vi "NumberStringConv.vi"() -> ()   [LabVIEW 2012]
panel:
  out "Complete?":bool
  out "(remainder string)":string
  out "Numeric (dbl)":dbl
  in  "String":string
  out "Numeric (String %#g with %p)":dbl
  out "Numeric (%g) 2":dbl
  out "Numeric (%#g) 2":dbl
  out "Numeric (%p) 2":dbl
  out "Numeric (%#p) 2":dbl
  out "Numeric (%g)":dbl
  out "Numeric (%#g)":dbl
  out "Numeric (%p)":dbl
  out "Numeric (%#p)":dbl
  out "String (%#g)":string
  out "String (%g)":string
  out "String (%p)":string
  out "String (%#p)":string
  in  "Numeric (dbl)":dbl
  # "Frac/Exp String to Number"
  # "Scan Value"
  # "Summary: %#p is a nice way to get compact notation, but it must be \nundone with ScanValue.vi and %p format (which handles e-notation)!"
  # "And as shown at the left, the %p format with Scan Value will still take a\nscientific notation string back to a double correctly!"
  # "Try any input in this box to validate the conversion.\n(see block diagram for method)."
  # "- Try m/u/k/M notation\n- try scientific notation\n- try garbage like 34e9g"
  # "Can check for any remainder string to see if \nentire string used to make number."
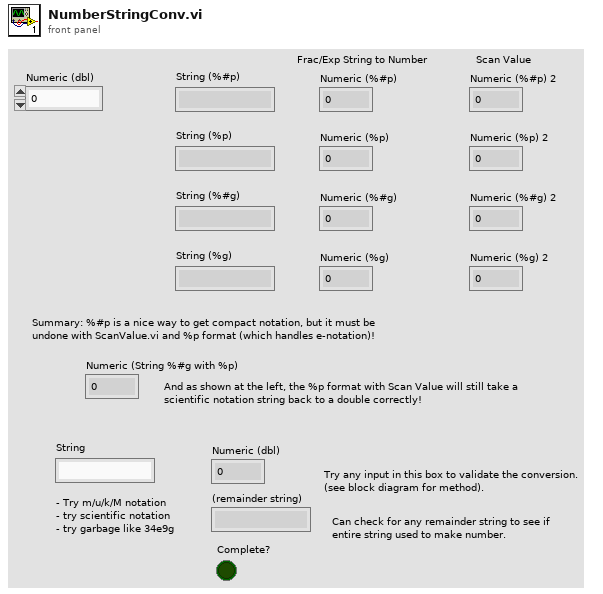
[diagram p1: front panel]
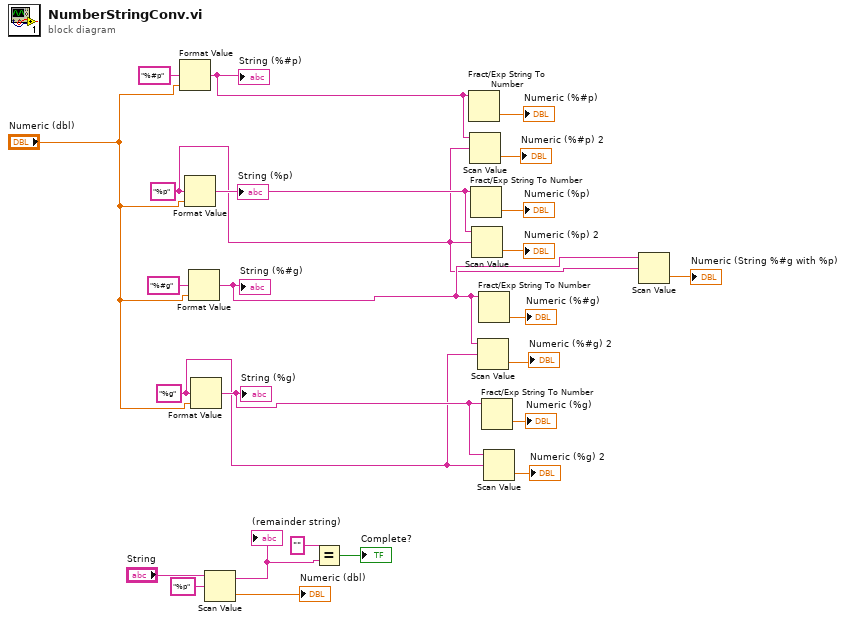
[diagram p0: block diagram]
diagram:
  w10 = "%g" ("format string")
  w7 = "%p" ("format string")
  n1 = Format Value(format string="%#p", value (0)="Numeric (dbl)") -> (output string=w15:string)  [unwired: 1 in]
  "String (%#p)" <- w15
  n2 = Format Value(format string=w7, value (0)="Numeric (dbl)") -> (output string=w14:string)  [unwired: 1 in]
  "String (%p)" <- w14
  n3 = Format Value(format string="%#g", value (0)="Numeric (dbl)") -> (output string=w8:string)  [unwired: 1 in]
  "String (%#g)" <- w8
  n4 = Format Value(format string=w10, value (0)="Numeric (dbl)") -> (output string=w13:string)  [unwired: 1 in]
  "String (%g)" <- w13
  n5 = Scan Value(string="String", format string="%p") -> (output string=w4:string, value=→"Numeric (dbl)":dbl)  [unwired: 1 in]
  "(remainder string)" <- w4
  n6 = Equal?(x="", y=w4) -> (x = y?=→"Complete?":bool)
  n7 = Fract/Exp String To Number(string=w15) -> (number=→"Numeric (%#p)":dbl)  [unwired: 3 in, 1 out]
  n8 = Scan Value(string=w15, format string=w7) -> (value=→"Numeric (%#p) 2":dbl)  [unwired: 1 in, 1 out]
  n9 = Fract/Exp String To Number(string=w14) -> (number=→"Numeric (%p)":dbl)  [unwired: 3 in, 1 out]
  n10 = Scan Value(string=w14, format string=w7) -> (value=→"Numeric (%p) 2":dbl)  [unwired: 1 in, 1 out]
  n11 = Scan Value(string=w8, format string=w10) -> (value=→"Numeric (%#g) 2":dbl)  [unwired: 1 in, 1 out]
  n12 = Fract/Exp String To Number(string=w8) -> (number=→"Numeric (%#g)":dbl)  [unwired: 3 in, 1 out]
  n13 = Fract/Exp String To Number(string=w13) -> (number=→"Numeric (%g)":dbl)  [unwired: 3 in, 1 out]
  n14 = Scan Value(string=w13, format string=w10) -> (value=→"Numeric (%g) 2":dbl)  [unwired: 1 in, 1 out]
  n15 = Scan Value(string=w8, format string=w7) -> (value=→"Numeric (String %#g with %p)":dbl)  [unwired: 1 in, 1 out]
